vi "Configure_PSG.vi"(2 "Power [dBm]":dbl=-130.0, 3 "Frequency [GHz]":dbl=100000.0, 4 "VISA resource name":refnum<visa-resource-name>="PSG1") -> ()   [LabVIEW 2011]
doc: "This example shows how to configure the frequency and power of the output signal."
uses:
  <instrlib>/Agilent PSG MXG Series/Agilent PSG MXG Series.lvlib
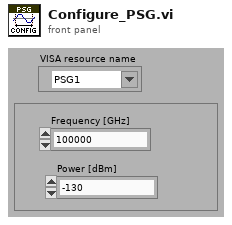
[diagram p1: front panel]
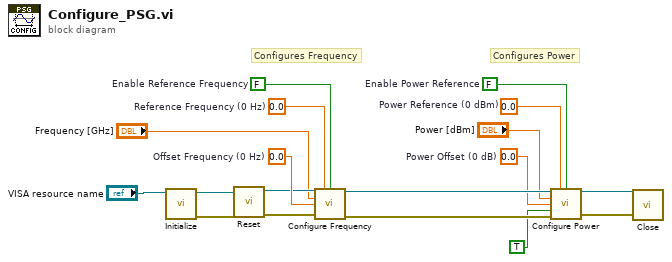
[diagram p0: block diagram]
diagram:
  w12 = 0.0  # Offset Frequency (0 Hz)
  w13 = 0.0  # Reference Frequency (0 Hz)
  w10 = 0.0  # Power Reference (0 dBm)
  w9 = 0.0  # Power Offset (0 dB)
  w11 = FALSE  # Enable Power Reference
  w14 = FALSE  # Enable Reference Frequency
  # "Configures Power"
  # "Configures Frequency"
  n1 = call <instrlib>:"Initialize.vi"("VISA resource name"="VISA resource name") -> ("error out"=w5:errorcluster, "VISA resource name out"=w7:refnum<visa-resource-name>)  [unwired: 9 in]
  n2 = call <instrlib>:"Reset.vi"("error in (no error)"=w5, "VISA resource name"=w7) -> ("error out"=w4:errorcluster, "VISA resource name out"=w6:refnum<visa-resource-name>)  [unwired: 8 in]
  n3 = call <instrlib>:"Configure Frequency.vi"("VISA resource name"=w6, "Reference Frequency (0 Hz)"=w13, "Enable Reference Frequency (F:Disable)"=w14, "Frequency (100 kHz)"="Frequency [GHz]", "Offset Frequency (0 Hz)"=w12, "error in (no error)"=w4) -> ("VISA resource name out"=w18:refnum<visa-resource-name>, "error out"=w17:errorcluster)  [unwired: 8 in]
  n4 = call <instrlib>:"Configure Power.vi"("VISA resource name"=w18, "Power Reference (0 dBm)"=w10, "Enable Power Reference (F:Disable)"=w11, "Power (-130 dBm)"="Power [dBm]", "Power Offset (0 dB)"=w9, "Attenuator Auto Mode (T:Enable)"=TRUE, "error in (no error)"=w17) -> ("VISA resource name out"=w2:refnum<visa-resource-name>, "error out"=w1:errorcluster)  [unwired: 7 in]
  n5 = call <instrlib>:"Close.vi"("error in (no error)"=w1, "VISA resource name"=w2) -> ()  [unwired: 9 in, 1 out]
